vi "Format.vi"(8 "error in (no error)":errorcluster, 10 "LogRecord":refnum<class "LogRecord.lvclass">, 11 "ILogFormatter in":refnum<class "ILogFormatter.lvclass">) -> (0 "error out":errorcluster, 2 "Log Line":string, 3 "ILogFormatter out":refnum<class "ILogFormatter.lvclass">)   [LabVIEW 2024, in "ILogFormatter.lvclass"]
uses:
  ILogFormatter.lvclass
  Record/LogRecord.lvclass
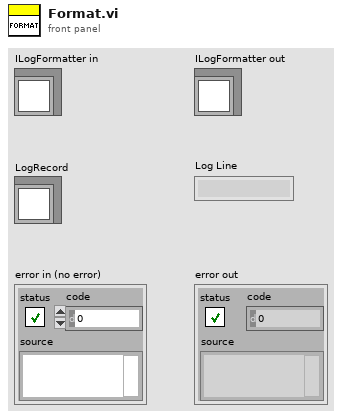
[diagram p1: front panel]
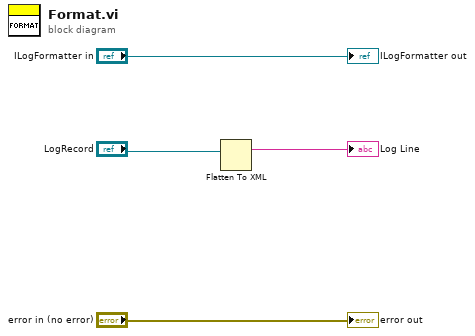
[diagram p0: block diagram]
diagram:
  n1 = Flatten To XML(6:"LogRecord") -> (2:→"Log Line":string)
  "error out" <- "error in (no error)"
  "ILogFormatter out" <- "ILogFormatter in"
